vi "GetStandardGap_Huan_21.07.2016.vi"(8 "Welcher Lautsprecher?":i32=13, 9 "Distance in dm":u8=13, 11 "Pfad-Datenbank":path=path "C:/Users/Administrator/Documents/New LabView Programms/Aktuelle Programme/Experiment!/HuanSubVIs/S70-21_M1.csv") -> (0 "Standard Gap":dbl, 3 "all rows":dbl[][](array[numeric])=[[0.0, 70.0, 80.0, 90.0, 100.0, 110.0, 120.0, 130.0, 140.0], [1.0, 72.09, 75.16, 75.91, 76.66, 77.68, 78.98, 78.81, 81.14], [2.0, 78.22, 79.36, 78.69, 80.06, 79.52, 85.61, 89.03, 89.56], [3.0, 81.87, 82.46, 83.33, 85.13, 82.83, 82.34, 82.96, 83.96], [4.0, 85.01, 84.72, 84.01, 83.17, 84.2, 84.58, 85.05, 85.48], [5.0, 82.85, 82.12, 83.29, 84.66, 82.16, 82.86, 83.93, 84.99], [6.0, 78.57, 78.98, 79.39, 80.47, 79.88, 82.41, 84.28, 84.79], [7.0, 73.84, 75.72, 77.0, 77.32, 78.31, 78.92, 79.31, 79.83], [8.0, 69.32, 71.56, 73.63, 74.82, 75.45, 76.25, 77.22, 77.55], [9.0, 66.75, 70.12, 71.47, 72.69, 73.97, 74.71, 75.22, 76.18], [10.0, 63.36, 66.68, 69.56, 71.12, 72.21, 73.57, 74.32, 74.31], [11.0, 62.06, 65.34, 67.97, 69.97, 71.3, 72.13, 0.0, 0.0], [12.0, 59.92, 63.2, 65.57, 67.4, 69.17, 69.85, 0.0, 0.0], [13.0, 60.94, 63.06, 64.92, 66.49, 68.11, 68.61, 0.0, 0.0], [14.0, 58.1, 61.01, 63.18, 0.0, 0.0, 0.0, 0.0, 0.0]] caption="Alle Zeilen" format="%0.3f")   [LabVIEW 2014]
uses:
  <vilib>/Utility/file.llb/Read From Spreadsheet File (DBL).vi
panel:
  out "x-y":u8=1
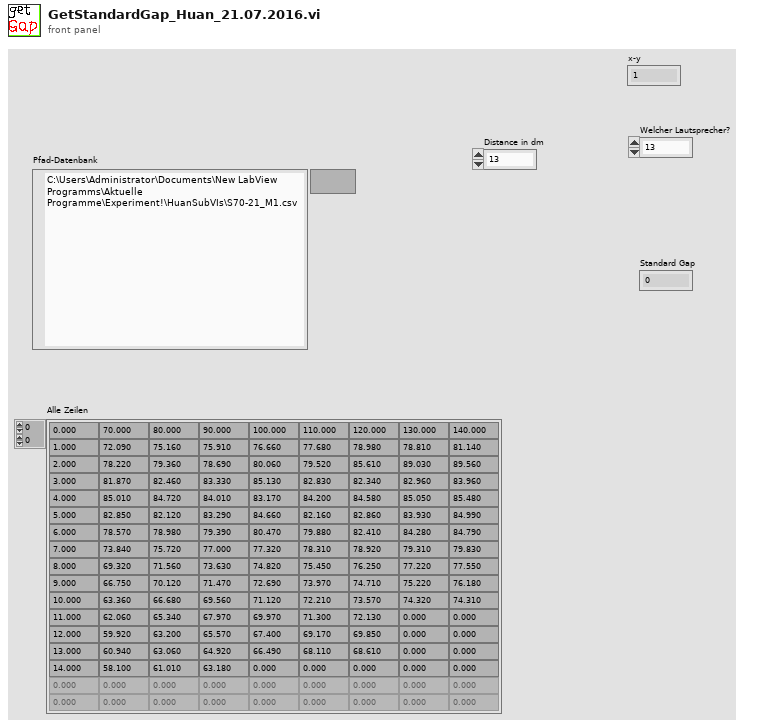
[diagram p1: front panel]
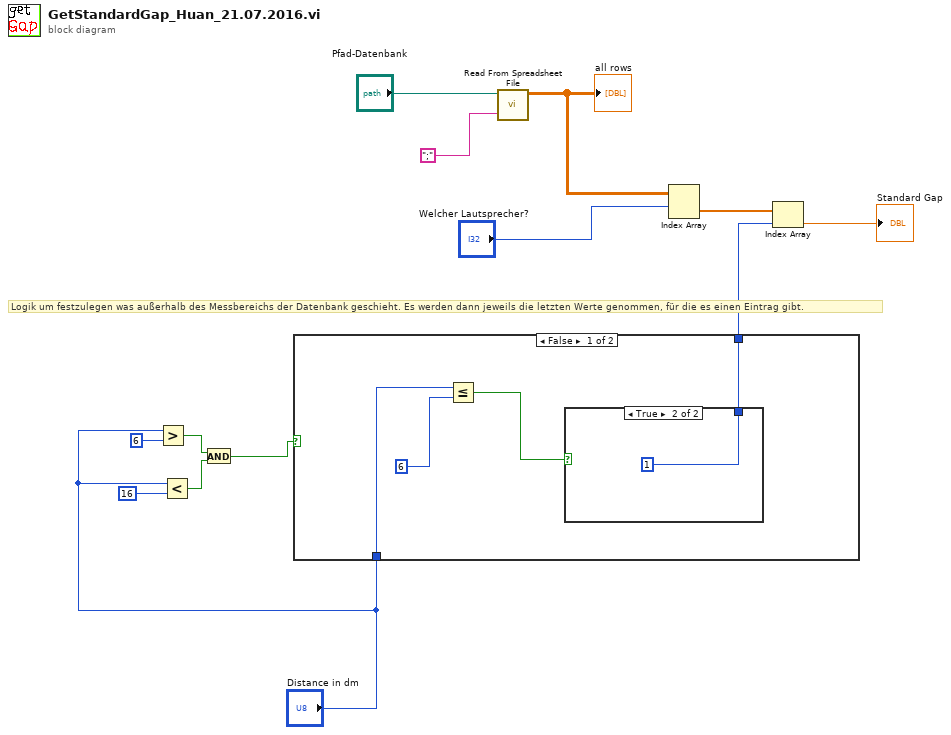
[diagram p0: block diagram]
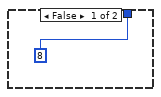
[diagram p2: hidden frame]
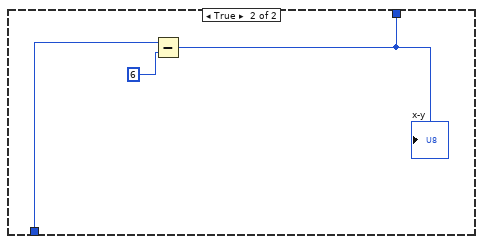
[diagram p3: hidden frame]
diagram:
  # "Logik um festzulegen was außerhalb des Messbereichs der Datenbank geschieht. Es werden dann jeweils die letzten Werte genommen, für die es einen Eintrag gibt."
  n1 = Greater?(x="Distance in dm", y=u8 6) -> (0:w4:bool)
  n2 = Less?(x="Distance in dm", y=u8 16) -> (x < y?=w3:bool)
  n3 = And(x=w4, y=w3) -> (x .and. y?=w2:bool)
  n4 = case shown="False" w2 {
    tunnel: "Distance in dm" -> [w16 w22]
    tunnel: [w17 w20] -> w8
    frame False {
      n5 = Less Or Equal?(x=w16, y=u8 6) -> (x <= y?=w14:bool)
      n6 = case shown="True" w14 {
        tunnel: [u8 8 u8 1] -> w17
        frame False {
        }
        frame True {
        }
      }
    }
    frame True {
      n7 = Subtract(x=w22, y=u8 6) -> (x-y=w20:u8)
      "x-y" <- w20
    }
  }
  n8 = call-poly <vilib>:"Read From Spreadsheet File.vi"("delimiter (\\t)"=";" ("delimiter (\\t)"), "file path (dialog if empty)"="Pfad-Datenbank") -> ("all rows"=w11:dbl[][])  [unwired: 5 in, 4 out]
  "all rows" <- w11
  n9 = Index Array(array=w11, index (row)="Welcher Lautsprecher?") -> (element=w9:dbl[])  [unwired: 1 in]
  n10 = Index Array(array=w9, index=w8) -> (element=→"Standard Gap":dbl)
